vi "inject-load-spikes.vi"(9 "inject-spikes":bool, 11 "Frequency and Amplitude In":T1={"frequency (Hz)"=60.0, "voltage (V) RMS"=1.0, "current (A) RMS"=1.0} {"current (A) RMS" scale=0.0..1.0; "voltage (V) RMS" scale=0.0..7.0; "frequency (Hz)" scale=40.0..60.0}) -> (3 "Frequency and Amplitude Out":T1={"frequency (Hz)"=60.0, "voltage (V) RMS"=1.0, "current (A) RMS"=1.0} {"current (A) RMS" scale=0.0..1.0; "voltage (V) RMS" scale=0.0..7.0; "frequency (Hz)" scale=40.0..60.0})   [LabVIEW 2024]
uses:
  <vilib>/numeric/Random Number (Range) DBL.vi
  <vilib>/ptbypt/NI_PtbyPt.lvlib
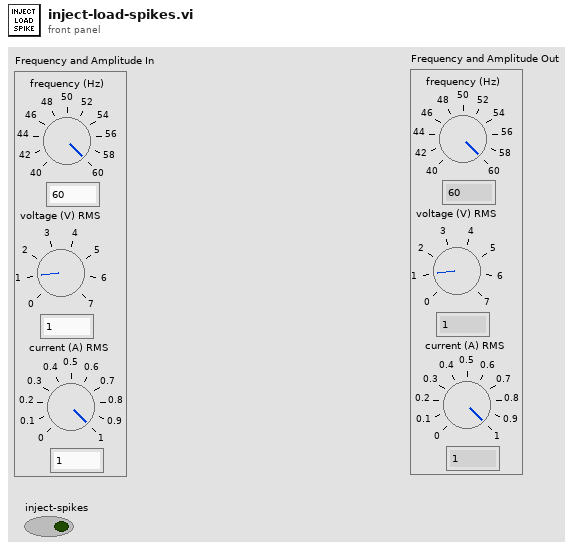
[diagram p1: front panel]
types:
  T1 = cluster{"frequency (Hz)":sgl, "voltage (V) RMS":dbl, "current (A) RMS":dbl}
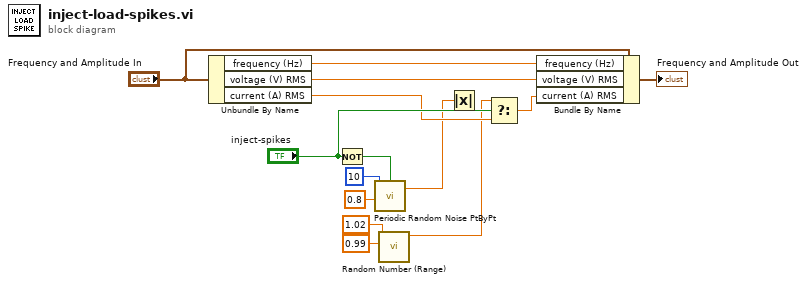
[diagram p0: block diagram]
diagram:
  n1 = Unbundle By Name("Frequency and Amplitude In") -> ("frequency (Hz)"=w11:sgl, "voltage (V) RMS"=w12:dbl, "current (A) RMS"=w5:dbl)
  n2 = Not(x="inject-spikes") -> (.not. x?=w6:bool)
  n3 = call <vilib>:"Periodic Random Noise PtByPt.vi"("initialize"=w6, "spectral amplitude"=0.8 ("standard deviation"), "sample length"=10) -> ("periodic random noise"=w4:dbl)  [unwired: 1 in, 1 out]
  n4 = call-poly <vilib>:"Random Number (Range).vi"("lower bound (0)"=0.99, "upper bound (100)"=1.02) -> ("number"=w3:dbl)  [unwired: 9 in]
  n5 = Absolute Value(x=w4) -> ()  [unwired: 1 out]
  n6 = Select(t=w3, s="inject-spikes", f=w5) -> (s? t:f=w9:dbl)
  n7 = Bundle By Name(cluster="Frequency and Amplitude In", "frequency (Hz)"=w11, "voltage (V) RMS"=w12, "current (A) RMS"=w9) -> (→"Frequency and Amplitude Out":T1)
